vi "DQMH Tester Cleanup hse-appl.vi"(8 "error in":errorcluster, 11 "Stop?":bool) -> (0 "error out":errorcluster)   [LabVIEW 2014, in "hse-dqmh.lvlib"]
doc: "If the hse-application object was instantiated and the hse-logger was initialized when starting the Tester, this VI cleans up both objects.\n\n____\nHAMPEL SOFTWARE ENGINEERING v0.7.0 (2018-07-16 18:12)"
uses:
  hse-dqmh.lvlib
  hse-application/hse-application.lvclass
  <vilib>/Hampel Software Engineering/HSE Logger/hse-logger.lvlib
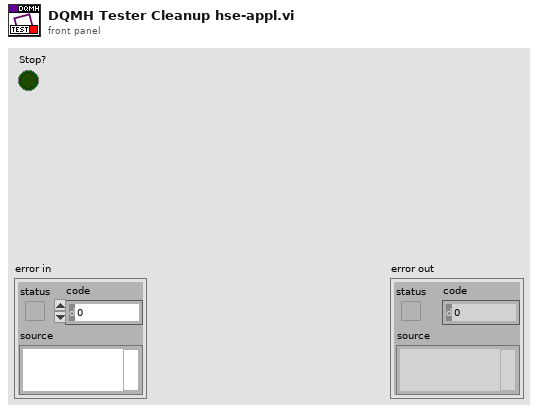
[diagram p1: front panel]
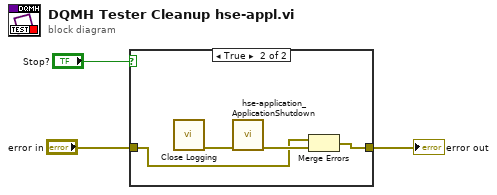
[diagram p0: block diagram]
diagram:
  n1 = case shown="True" "Stop?" {
    tunnel: "error in" -> [w4 w6]
    tunnel: [w4 w7] -> w2
    frame False {
    }
    frame True {
      n2 = call <vilib>:"Close Logging.vi"() -> ("error out"=w5:errorcluster)  [unwired: 11 in]
      n3 = call "hse-application_ApplicationShutdown.vi"("error in"=w5) -> ("error out"=w8:errorcluster)  [unwired: 10 in]
      n4 = Merge Errors(w6, w8) -> (w7:errorcluster)
    }
  }
  "error out" <- w2
